vi "Unit vector_3Dpf.vi"(0 "Vector":sgl[](array[numeric])) -> (1 "Unit vector":sgl[](array[numeric]), 2 "Vector magnitude":sgl)   [LabVIEW 2017]
panel:
  # "PN 13/01/2015"
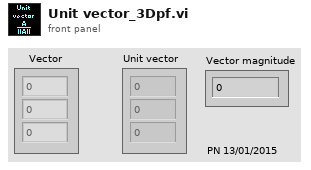
[diagram p1: front panel]
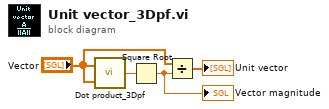
[diagram p0: block diagram]
diagram:
  n1 = call "Dot product_3Dpf.vi"("B"="Vector", "A"="Vector") -> ("A . B"=w4:sgl)
  n2 = Square Root(x=w4) -> (sqrt(x)=w1:sgl)
  "Vector magnitude" <- w1
  n3 = Divide(x="Vector", y=w1) -> (x/y=→"Unit vector":sgl[])
